vi "Generate Path from String Array.vi"(10 "String Array":string[](array[string]), 11 "Base Path":path) -> (3 "project folder out":path)   [LabVIEW 2019]
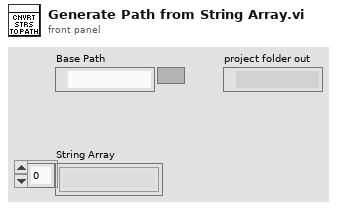
[diagram p1: front panel]
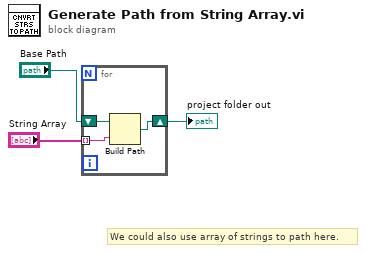
[diagram p0: block diagram]
diagram:
  # "We could also use array of strings to path here."
  n1 = for {
    shift-right: [w4] -> w3
    shift-left: "Base Path" -> [w5]
    tunnel: "String Array" -> [w6] mode=indexing
    n2 = Build Path(base path=w5, name or relative path=w6) -> (appended path=w4:path)
  }
  "project folder out" <- w3
